vi "Autonomous Independent.vi"() -> ()   [LabVIEW 2012]
doc: "This VI is called when autonomous begins, and will automatically be terminated when autonomous ends. You can carry out timed or sensor driven robot movement independently without needing to return to the caller."
uses:
  <vilib>/Rock Robotics/WPI/SafetyOutput/WPI_SafetyOutputConfigMenu.ctl
  <vilib>/Rock Robotics/WPI/DriverStation/DriverStationLCD/WPI_DriverStationLCDLCDLine.ctl
  <vilib>/Rock Robotics/WPI/Solenoid/WPI_SolenoidValue.ctl
  <vilib>/Rock Robotics/WPI/RobotDrive/WPI_RobotDriveGetSetRefNum.vi
  <vilib>/Rock Robotics/WPI/Solenoid/WPI_SolenoidSetEnum.vi
  Robot Global Data.vi
  <vilib>/Rock Robotics/WPI/Joystick/WPI_JoystickGetSetRefNum.vi
  <vilib>/Rock Robotics/WPI/RobotDrive/WPI_RobotDriveArcadeDrive_Standard(NoSaturation).vi
panel:
  in  "Array of robot movements 2":T1(array[cluster]) {"Y Joystick Value" scale=1.0..-1.0; "X Joystick Value" scale=-1.0..1.0}
  out "Current Movement, for debugging 2":T2 {"Y Joystick Value" scale=1.0..-1.0; "X Joystick Value" scale=-1.0..1.0}
  out "Current Movement, for debugging":T2 {"Y Joystick Value" scale=1.0..-1.0; "X Joystick Value" scale=-1.0..1.0}
  in  "Array of robot movements":T1(array[cluster]) {"Y Joystick Value" scale=1.0..-1.0; "X Joystick Value" scale=-1.0..1.0}
  # "Be sure to right-click and choose Data Operations>>Make Current Value default if you want to save the array values with the VI"
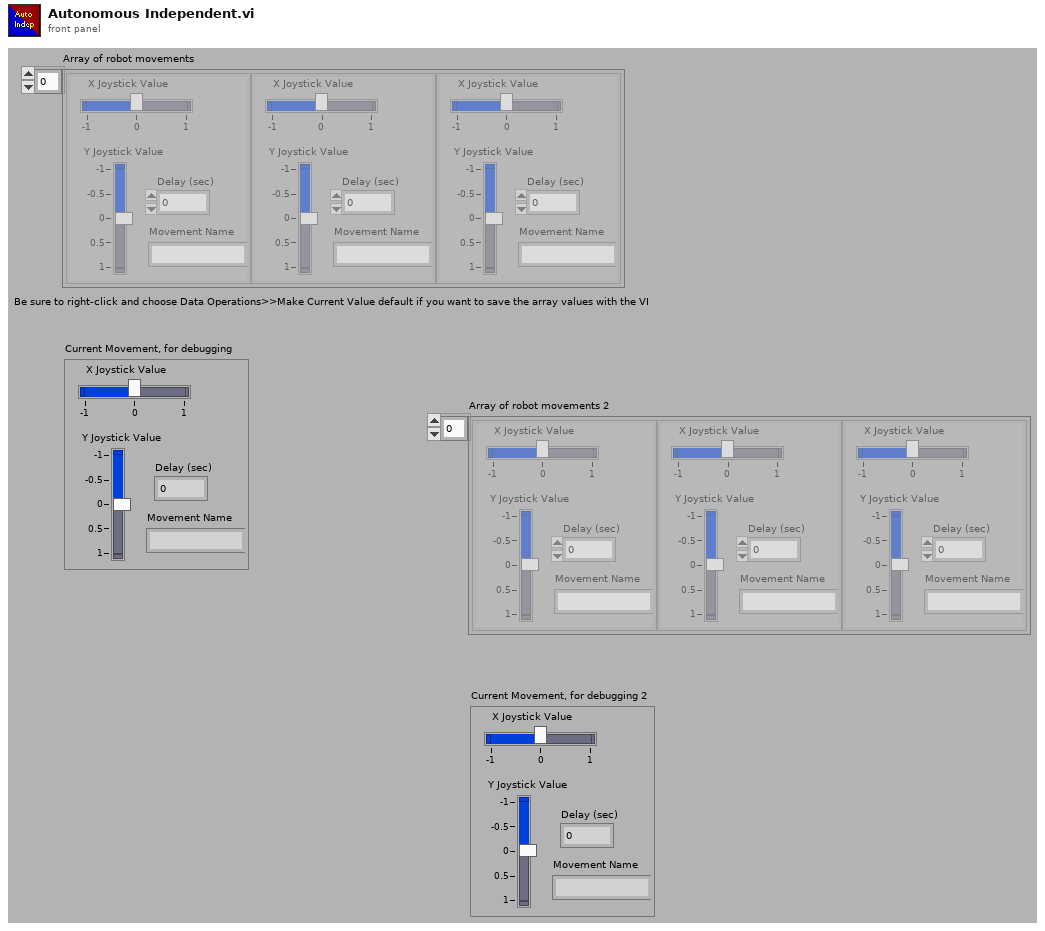
[diagram p1: front panel]
types:
  T1 = cluster{"X Joystick Value":dbl, "Y Joystick Value":dbl, "Delay (sec)":dbl, "Movement Name":string}[]
  T2 = cluster{"X Joystick Value":dbl, "Y Joystick Value":dbl, "Delay (sec)":dbl, "Movement Name":string}
  T3 = typedef "WPI_RobotDriveDevRef.ctl" = cluster{"DevStatus":errorcluster, "Motors[]":T4[], "Square Inputs":bool, "Max Output":dbl, "Isochronous":bool}
  T4 = typedef "WPI_MotorControlDeviceRef.ctl" = cluster{"DeviceStatus":errorcluster, "Type":enum16{"PWM", "CAN"}, "PWM":cluster{"Digital Module":T5, "PWM Channel":T6, "DeadBand":T7}, "CAN":cluster{"Device Number":u8, "Control Mode":T8, "Semaphore":T9, "Max Vout":dbl}, "Invert":bool, "TransformRef":T10, "InvTransformRef":T10}
  T5 = typedef "FPGA_TypedefDigitalModule.ctl" = enum16{"Digital Module 1", "Digital Module 2"}
  T6 = typedef "FPGA_DIOPWMChannel.ctl" = enum8{"PWM 1", "PWM 2", "PWM 3", "PWM 4", "PWM 5", "PWM 6", "PWM 7", "PWM 8", "PWM 9", "PWM 10", "Invalid"}
  T7 = typedef "WPI_PWMDeadband.ctl" = cluster{"Name":string, "maxPositivePwm":i32, "minPositivePwm":i32, "centerPwm":i32, "maxNegativePwm":i32, "minNegativePwm":i32, "angularRange":u16}
  T8 = typedef "WPI_CANJaguar_ControlMode.ctl" = enum8{"Percent VBus", "Current", "Speed", "Position", "Voltage"}
  T9 = typedef "Semaphore RefNum" = refnum<k1>
  T10 = typedef "WPI_PWMTransform_ConPane.ctl" = refnum<vi>
  T11 = typedef "WPI_JoystickDevRef.ctl" = cluster{"Device":T12}
  T12 = typedef "WPI_JoystickDeviceEnum.ctl" = enum16{"USB 1", "USB 2", "USB 3", "USB 4", "Kinect 1", "Kinect 2"}
  T13 = cluster{"axis 1 (x)":dbl, "axis 2 (y)":dbl, "axis 3 (throttle)":dbl, "axis 4":dbl, "axis 5":dbl, "axis 6":dbl}
  T14 = typedef "WPI_DriverStationLCDLCDLine.ctl" = enum16{"Main - Line 1", "User - Line 2", "User - Line 3", "User - Line 4", "User - Line 5", "User - Line 6"}
  T15 = typedef "WPI_SafetyOutputConfigMenu.ctl" = enum16{"Enable", "Disable"}
  T16 = typedef "WPI_SolenoidValue.ctl" = enum16{"Off", "On", "Forward", "Reverse"}
  T17 = typedef "WPI_SolenoidDevRef.ctl" = cluster{"DevStatus":errorcluster, "Solenoid Module":T18, "Forward Solenoid Channel":T19, "Reverse Solenoid Channel":T19}
  T18 = typedef "FPGA_TypedefSolenoidModule.ctl" = enum16{"Solenoid Module 1", "Solenoid Module 2"}
  T19 = typedef "WPI_SolenoidChannel.ctl" = enum8{"Solenoid 1", "Solenoid 2", "Solenoid 3", "Solenoid 4", "Solenoid 5", "Solenoid 6", "Solenoid 7", "Solenoid 8", "Invalid"}
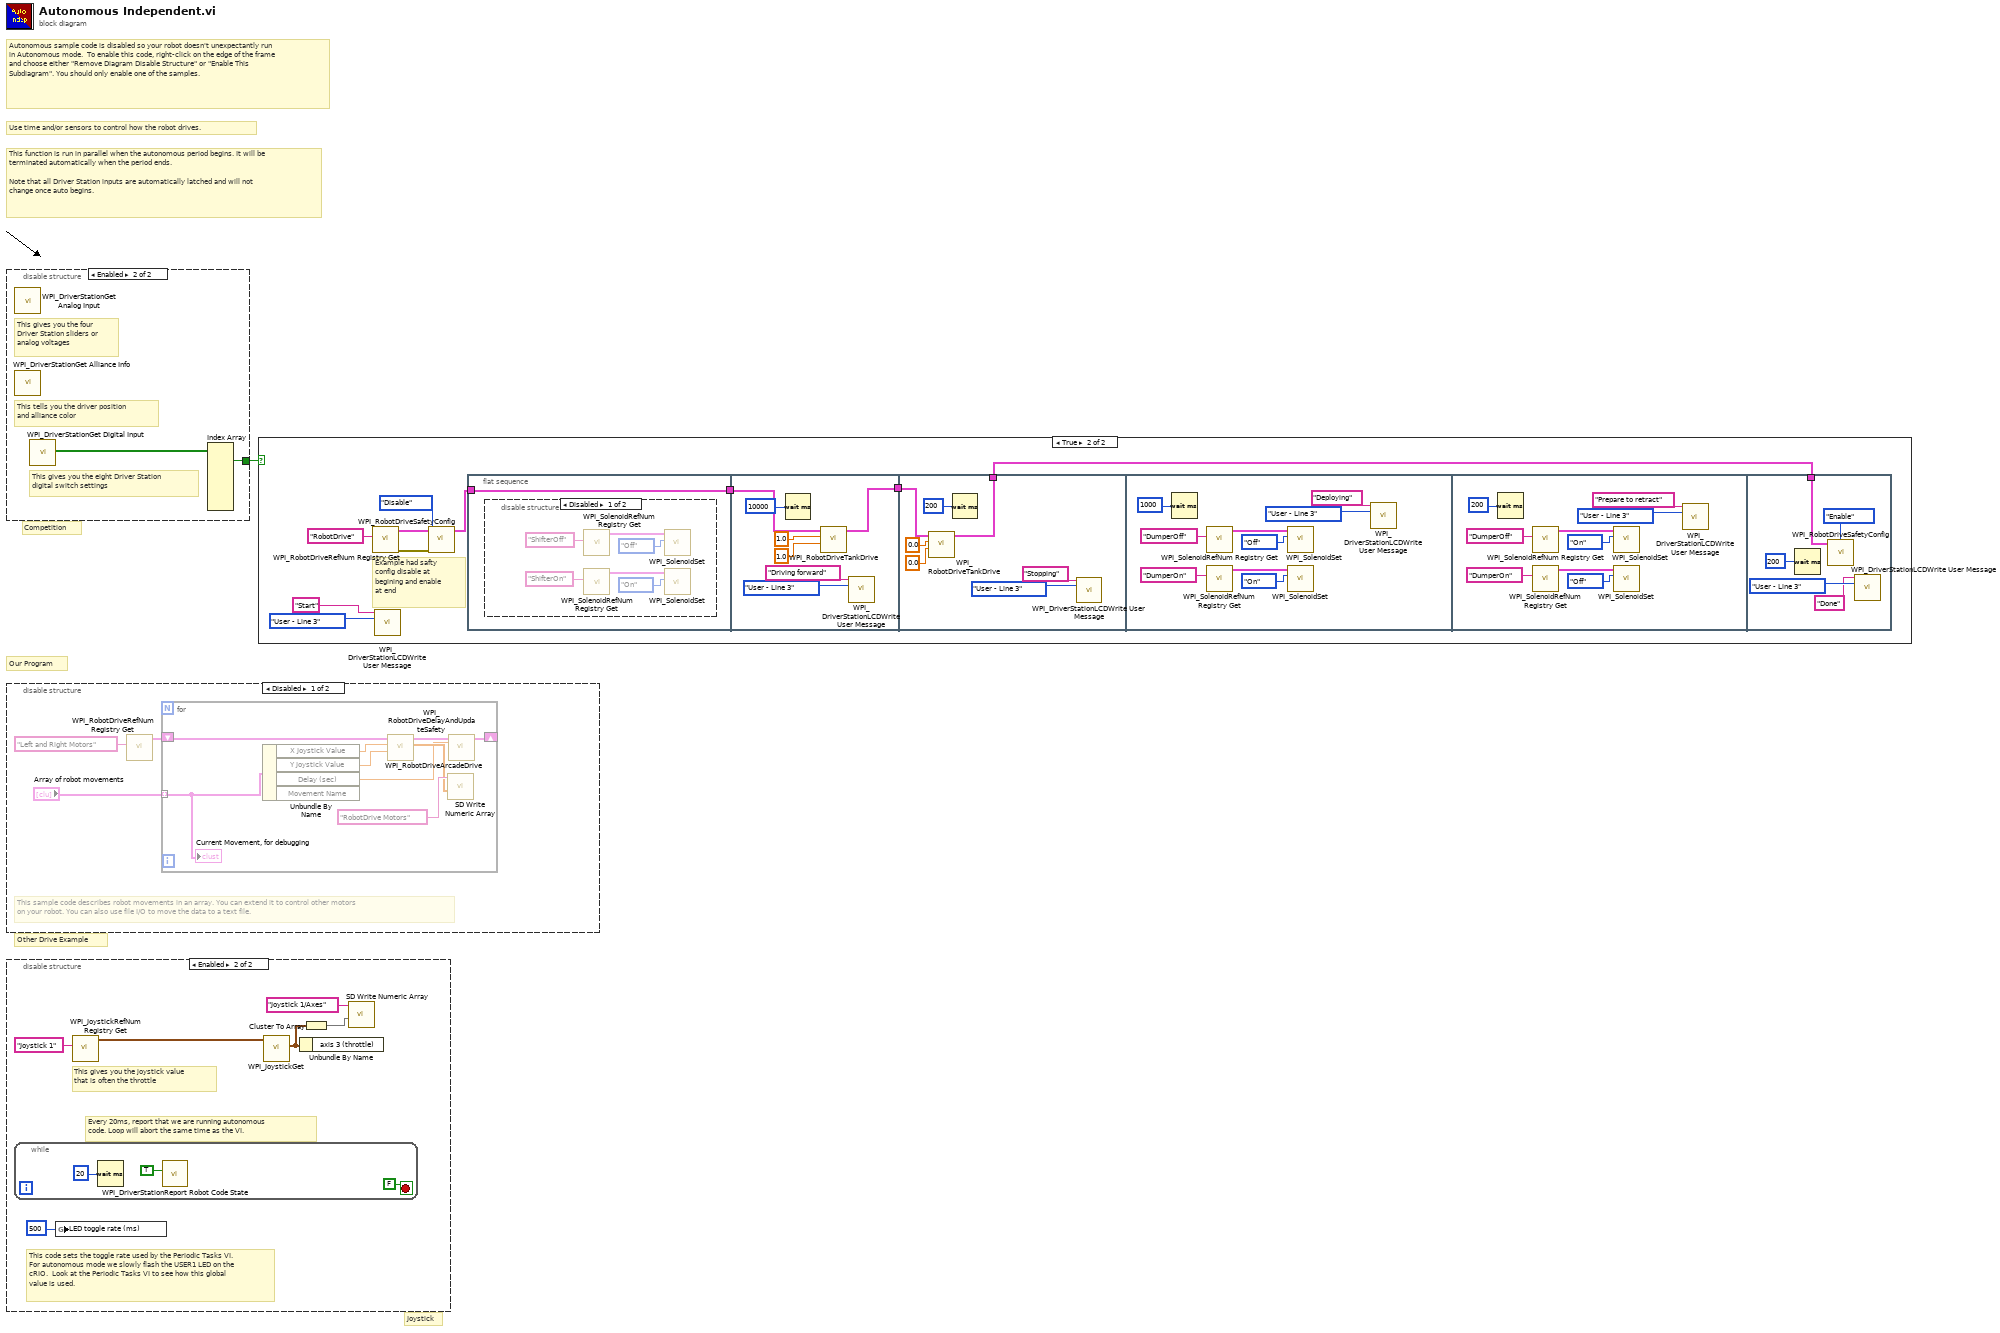
[diagram p0: block diagram]
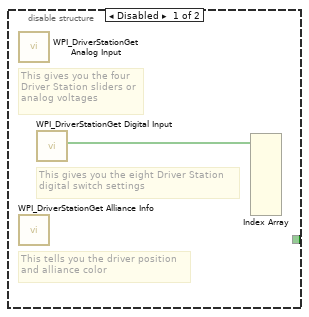
[diagram p4: hidden frame]
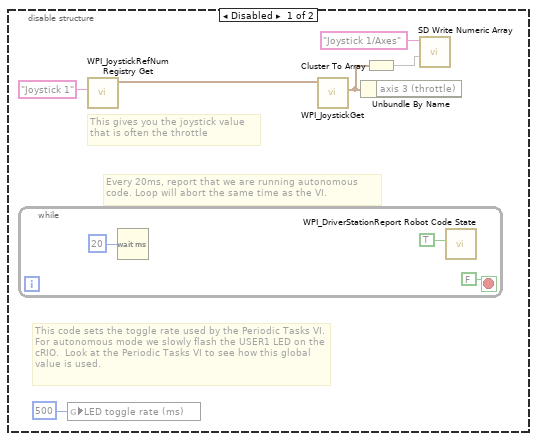
[diagram p5: hidden frame]
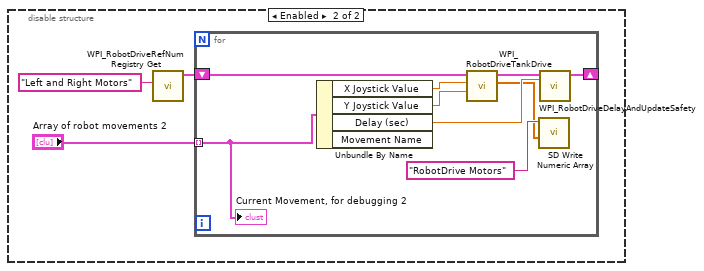
[diagram p6: hidden frame]
diagram:
  # "Our Program"
  # "Autonomous sample code is disabled so your robot doesn't unexpectantly run in Autonomous mode.  To enable this code, right-click on the edge of the frame and choose either \"Remove Diagram Disable Structure\" or \"Enable This Subdiagram\". You should only enable one of the samples."
  # "This function is run in parallel when the autonomous period begins. It will be terminated automatically when the period ends.\n\nNote that all Driver Station inputs are automatically latched and will not change once auto begins."
  # "Joystick"
  # "Competition"
  # "Other Drive Example"
  # "Use time and/or sensors to control how the robot drives."
  n1 = disable-structure shown="Enabled" {
    disable-tunnel: [_ w3] -> w1
    frame Disabled {
      # "This tells you the driver position\nand alliance color"
      # "This gives you the eight Driver Station\ndigital switch settings"
      # "This gives you the four\nDriver Station sliders or\nanalog voltages"
      n2 = call <vilib>:"WPI_DriverStationGet Analog Input.vi"() -> ()  [unwired: 12 out]
      n3 = call <vilib>:"WPI_DriverStationGet Alliance Info.vi"() -> ()  [unwired: 12 out]
      n4 = call <vilib>:"WPI_DriverStationGet Digital Input.vi"() -> ("Driver Station Digital Input (1-8)"=w2:bool[])  [unwired: 11 out]
      n5 = Index Array(array=w2) -> ()  [unwired: 8 in, 8 out]
    }
    frame Enabled {
      # "This tells you the driver position\nand alliance color"
      # "This gives you the eight Driver Station\ndigital switch settings"
      # "This gives you the four\nDriver Station sliders or\nanalog voltages"
      n6 = call <vilib>:"WPI_DriverStationGet Analog Input.vi"() -> ()  [unwired: 12 out]
      n7 = call <vilib>:"WPI_DriverStationGet Alliance Info.vi"() -> ()  [unwired: 12 out]
      n8 = call <vilib>:"WPI_DriverStationGet Digital Input.vi"() -> ("Driver Station Digital Input (1-8)"=w4:bool[])  [unwired: 11 out]
      n9 = Index Array(array=w4) -> (element #1=w3:bool)  [unwired: 8 in, 7 out]
    }
  }
  n10 = disable-structure shown="Disabled" {
    frame Disabled {
      # "This sample code describes robot movements in an array. You can extend it to control other motors\non your robot. You can also use file I/O to move the data to a text file."
      n11 = call <vilib>:"WPI_RobotDriveRefNum Registry Get.vi"("refnum name"="Left and Right Motors") -> ("RobotDriveDevRef"=w6:T3)  [unwired: 1 in, 9 out]
      n12 = for {
        shift-right: [w12] -> _
        shift-left: w6 -> [w13]
        tunnel: "Array of robot movements" -> [w8] mode=indexing
        n13 = Unbundle By Name(w8) -> ("X Joystick Value"=w11:dbl, "Y Joystick Value"=w10:dbl, "Delay (sec)"=w9:dbl)  [unwired: 1 out]
        n14 = call-poly <vilib>:"WPI_RobotDriveArcadeDrive.vi"("Y axis value"=w10, "X axis value"=w11, "RobotDriveDevRef"=w13) -> ("Motor Values"=w15:dbl[], "RobotDriveDevRef"=w14:T3)  [unwired: 1 in, 6 out]
        n15 = call <vilib>:"SD Write Numeric Array.vi"("Numeric Array"=w15, "Name"="RobotDrive Motors") -> ()  [unwired: 8 in, 2 out]
        n16 = call <vilib>:"WPI_RobotDriveDelayAndUpdateSafety.vi"("Delay (s)"=w9, "RobotDriveDevRef"=w14) -> ("RobotDriveDevRef 2"=w12:T3)  [unwired: 8 in, 1 out]
        "Current Movement, for debugging" <- w8
      }
    }
    frame Enabled {
      n17 = call <vilib>:"WPI_RobotDriveRefNum Registry Get.vi"("refnum name"="Left and Right Motors") -> ("RobotDriveDevRef"=w18:T3)  [unwired: 1 in, 9 out]
      n18 = for {
        shift-right: [w27] -> _
        shift-left: w18 -> [w20]
        tunnel: "Array of robot movements 2" -> [w25] mode=indexing
        n19 = Unbundle By Name(w25) -> ("X Joystick Value"=w24:dbl, "Y Joystick Value"=w23:dbl, "Delay (sec)"=w26:dbl)  [unwired: 1 out]
        n20 = call <vilib>:"WPI_RobotDriveTankDrive.vi"("Right axis value"=w23, "Left axis value"=w24, "RobotDriveDevRef"=w20) -> ("Motor Values"=w22:dbl[], "RobotDriveDevRef"=w21:T3)  [unwired: 6 in, 1 out]
        n21 = call <vilib>:"SD Write Numeric Array.vi"("Numeric Array"=w22, "Name"="RobotDrive Motors") -> ()  [unwired: 8 in, 2 out]
        n22 = call <vilib>:"WPI_RobotDriveDelayAndUpdateSafety.vi"("Delay (s)"=w26, "RobotDriveDevRef"=w21) -> ("RobotDriveDevRef 2"=w27:T3)  [unwired: 8 in, 1 out]
        "Current Movement, for debugging 2" <- w25
      }
    }
  }
  n23 = disable-structure shown="Enabled" {
    frame Disabled {
      # "This code sets the toggle rate used by the Periodic Tasks VI.  For autonomous mode we slowly flash the USER1 LED on the cRIO.  Look at the Periodic Tasks VI to see how this global value is used."
      # "Every 20ms, report that we are running autonomous\ncode. Loop will abort the same time as the VI."
      # "This gives you the joystick value\nthat is often the throttle"
      n24 = while {
        stop <- FALSE stop-if-true
        n25 = Wait (ms)(milliseconds to wait=u32 20) -> ()  [unwired: 1 out]
        n26 = call <vilib>:"WPI_DriverStationReport Robot Code State.vi"("Autonomous"=TRUE) -> ()  [unwired: 10 in, 1 out]
      }
      n27 = global write "Robot Global Data.vi" "LED toggle rate (ms)"(u32 500 ("LED ms toggle rate")) -> ()
      n28 = call <vilib>:"WPI_JoystickRefNum Registry Get.vi"("refnum name"="Joystick 1") -> ("JoystickDevRef"=w33:T11)  [unwired: 1 in, 9 out]
      n29 = call <vilib>:"WPI_JoystickGet.vi"("JoystickDevRef"=w33) -> ("Axes"=w30:T13)  [unwired: 1 in, 5 out]
      n30 = Unbundle By Name(w30) -> ()  [unwired: 1 out]
      n31 = Cluster To Array(cluster=w30) -> (array=w31:dbl[])
      n32 = call <vilib>:"SD Write Numeric Array.vi"("Numeric Array"=w31, "Name"="Joystick 1/Axes") -> ()  [unwired: 8 in, 2 out]
    }
    frame Enabled {
      # "This code sets the toggle rate used by the Periodic Tasks VI.  For autonomous mode we slowly flash the USER1 LED on the cRIO.  Look at the Periodic Tasks VI to see how this global value is used."
      # "Every 20ms, report that we are running autonomous\ncode. Loop will abort the same time as the VI."
      # "This gives you the joystick value\nthat is often the throttle"
      n33 = while {
        stop <- FALSE stop-if-true
        n34 = Wait (ms)(milliseconds to wait=u32 20) -> ()  [unwired: 1 out]
        n35 = call <vilib>:"WPI_DriverStationReport Robot Code State.vi"("Autonomous"=TRUE) -> ()  [unwired: 10 in, 1 out]
      }
      n36 = global write "Robot Global Data.vi" "LED toggle rate (ms)"(u32 500 ("LED ms toggle rate")) -> ()
      n37 = call <vilib>:"WPI_JoystickRefNum Registry Get.vi"("refnum name"="Joystick 1") -> ("JoystickDevRef"=w40:T11)  [unwired: 1 in, 9 out]
      n38 = call <vilib>:"WPI_JoystickGet.vi"("JoystickDevRef"=w40) -> ("Axes"=w43:T13)  [unwired: 1 in, 5 out]
      n39 = Unbundle By Name(w43) -> ()  [unwired: 1 out]
      n40 = Cluster To Array(cluster=w43) -> (array=w42:dbl[])
      n41 = call <vilib>:"SD Write Numeric Array.vi"("Numeric Array"=w42, "Name"="Joystick 1/Axes") -> ()  [unwired: 8 in, 2 out]
    }
  }
  n42 = case shown="True" w1 {
    frame False {
    }
    frame True {
      # "Example had safty\nconfig disable at \nbegining and enable\nat end"
      n43 = call <vilib>:"WPI_RobotDriveRefNum Registry Get.vi"("refnum name"="RobotDrive" ("Name")) -> ("error out"=w52:errorcluster, "RobotDriveDevRef"=w55:T3)  [unwired: 1 in, 8 out]
      n44 = call <vilib>:"WPI_DriverStationLCDWrite User Message.vi"("line text"="Start", "line"=WPI_DriverStationLCDLCDLine."User - Line 3") -> ()  [unwired: 13 in, 1 out]
      n45 = call <vilib>:"WPI_RobotDriveSafetyConfig.vi"("error in (no error)"=w52, "mode"=WPI_SafetyOutputConfigMenu."Disable", "RobotDriveDevRef"=w55) -> ("RobotDriveDevRef"=w54:T3)  [unwired: 7 in, 1 out]
      n46 = flat-sequence {
        tunnel: w54 -> [w57]
        tunnel: [w57] -> w48
        tunnel: [w66] -> w47
        tunnel: w48 -> [w70]
        tunnel: w47 -> [w74]
        tunnel: [w73] -> w51
        tunnel: w51 -> [w100]
        frame #0 {
          n47 = disable-structure shown="Disabled" {
            frame Disabled {
              n48 = call <vilib>:"WPI_SolenoidRefNum Registry Get.vi"("refnum name"="ShifterOff") -> ("SolenoidDevRef"=w62:T17)  [unwired: 9 in, 1 out]
              n49 = call <vilib>:"WPI_SolenoidRefNum Registry Get.vi"("refnum name"="ShifterOn") -> ("SolenoidDevRef"=w63:T17)  [unwired: 9 in, 1 out]
              n50 = call-poly <vilib>:"WPI_SolenoidSet.vi"("Value"=WPI_SolenoidValue."Off", "SolenoidDevRef"=w62) -> ()  [unwired: 8 in, 2 out]
              n51 = call-poly <vilib>:"WPI_SolenoidSet.vi"("Value"=WPI_SolenoidValue."On", "SolenoidDevRef"=w63) -> ()  [unwired: 8 in, 2 out]
            }
            frame Enabled {
            }
          }
        }
        frame #1 {
          n52 = Wait (ms)(milliseconds to wait=u32 10000) -> ()  [unwired: 1 out]
          n53 = call <vilib>:"WPI_RobotDriveTankDrive.vi"("Right axis value"=1.0, "Left axis value"=1.0, "RobotDriveDevRef"=w70) -> ("RobotDriveDevRef"=w66:T3)  [unwired: 6 in, 2 out]
          n54 = call <vilib>:"WPI_DriverStationLCDWrite User Message.vi"("line text"="Driving forward", "line"=WPI_DriverStationLCDLCDLine."User - Line 3") -> ()  [unwired: 13 in, 1 out]
        }
        frame #2 {
          n55 = call <vilib>:"WPI_RobotDriveTankDrive.vi"("Right axis value"=0.0, "Left axis value"=0.0, "RobotDriveDevRef"=w74) -> ("RobotDriveDevRef"=w73:T3)  [unwired: 6 in, 2 out]
          n56 = Wait (ms)(milliseconds to wait=u32 200) -> ()  [unwired: 1 out]
          n57 = call <vilib>:"WPI_DriverStationLCDWrite User Message.vi"("line text"="Stopping", "line"=WPI_DriverStationLCDLCDLine."User - Line 3") -> ()  [unwired: 13 in, 1 out]
        }
        frame #3 {
          n58 = Wait (ms)(milliseconds to wait=u32 1000) -> ()  [unwired: 1 out]
          n59 = call <vilib>:"WPI_SolenoidRefNum Registry Get.vi"("refnum name"="DumperOff") -> ("SolenoidDevRef"=w81:T17)  [unwired: 9 in, 1 out]
          n60 = call <vilib>:"WPI_SolenoidRefNum Registry Get.vi"("refnum name"="DumperOn") -> ("SolenoidDevRef"=w80:T17)  [unwired: 9 in, 1 out]
          n61 = call-poly <vilib>:"WPI_SolenoidSet.vi"("Value"=WPI_SolenoidValue."Off", "SolenoidDevRef"=w81) -> ()  [unwired: 8 in, 2 out]
          n62 = call-poly <vilib>:"WPI_SolenoidSet.vi"("Value"=WPI_SolenoidValue."On", "SolenoidDevRef"=w80) -> ()  [unwired: 8 in, 2 out]
          n63 = call <vilib>:"WPI_DriverStationLCDWrite User Message.vi"("line text"="Deploying", "line"=WPI_DriverStationLCDLCDLine."User - Line 3") -> ()  [unwired: 13 in, 1 out]
        }
        frame #4 {
          n64 = Wait (ms)(milliseconds to wait=u32 200) -> ()  [unwired: 1 out]
          n65 = call <vilib>:"WPI_SolenoidRefNum Registry Get.vi"("refnum name"="DumperOff") -> ("SolenoidDevRef"=w90:T17)  [unwired: 9 in, 1 out]
          n66 = call <vilib>:"WPI_SolenoidRefNum Registry Get.vi"("refnum name"="DumperOn") -> ("SolenoidDevRef"=w89:T17)  [unwired: 9 in, 1 out]
          n67 = call-poly <vilib>:"WPI_SolenoidSet.vi"("Value"=WPI_SolenoidValue."On", "SolenoidDevRef"=w90) -> ()  [unwired: 8 in, 2 out]
          n68 = call-poly <vilib>:"WPI_SolenoidSet.vi"("Value"=WPI_SolenoidValue."Off", "SolenoidDevRef"=w89) -> ()  [unwired: 8 in, 2 out]
          n69 = call <vilib>:"WPI_DriverStationLCDWrite User Message.vi"("line text"="Prepare to retract", "line"=WPI_DriverStationLCDLCDLine."User - Line 3") -> ()  [unwired: 13 in, 1 out]
        }
        frame #5 {
          n70 = Wait (ms)(milliseconds to wait=u32 200) -> ()  [unwired: 1 out]
          n71 = call <vilib>:"WPI_RobotDriveSafetyConfig.vi"("mode"=WPI_SafetyOutputConfigMenu."Enable", "RobotDriveDevRef"=w100) -> ()  [unwired: 8 in, 2 out]
          n72 = call <vilib>:"WPI_DriverStationLCDWrite User Message.vi"("line text"="Done", "line"=WPI_DriverStationLCDLCDLine."User - Line 3") -> ()  [unwired: 13 in, 1 out]
        }
      }
    }
  }
